vi "Game Controller.vi"(8 "error in (no error)":errorcluster, 9 "Direction":T1, 11 "Application in":refnum<class "Game.lvclass">) -> (0 "error out":errorcluster, 3 "Application out":refnum<class "Game.lvclass">)   [LabVIEW 2021, in "Game.lvclass"]
doc: "Handles the logic process to respawn, manage and control all elements that appear in the board game"
uses:
  Game.lvclass
  GameEl_class/private/Enum Direction.ctl
  Game.lvclass/Game.ctl
  Imposible_Snake_v2/LVApp/Modules/Sound Manager/Typedefs/Sound Effects.ctl
  Board Game_class/Board Game.lvclass
  Imposible_Snake_v2/LVApp/Modules/Sound Manager/Sound Manager.lvlib
  GameEl_class/GameEl.lvclass
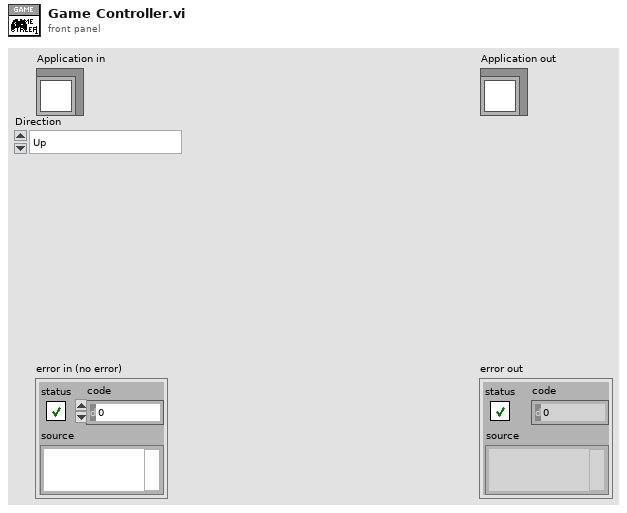
[diagram p1: front panel]
types:
  T1 = typedef "GameEl.lvclass/Enum Direction.ctl" = enum16{"Up", "Down", "Forward", "Backward"}
  T2 = typedef "Sound Manager.lvlib/Sound Effects.ctl" = enum16{"Bomb In", "Bomb Out", "Bomb Touched", "Game Over", "Victory", "Eat", "10 Fruits", "Eat2", "Eat3", "Eat4", "MaxShield", "Shield", "10p", "Grape In", "Grape Out", "20p", "30p", "40p", "50p", "60p", "70p", "80p", "90p", "100p", "All shields cracked", "Mouse In", "Mouse Out", "Mouse Eaten", "Grape Eaten", "States Recover", "Broken Shield", "Bonus", "Happy Time", "explode", "Game over musica", "Back Music", "Shield Catch", "Evil lough", "Cricket In", "Cricket eaten", "Lets Go", "Jump1", "Jump2", "Jump3", "Unstoppable", "Troll Music", "winner", "menu"}
  T3 = typedef "Game.lvclass/Packed Refs.ctl" = cluster{"graphics queue":refnum<queue>, "Stop Control Loop":refnum<user-event>, "Direction":refnum<notifier>, "Timer":refnum<data-value>}
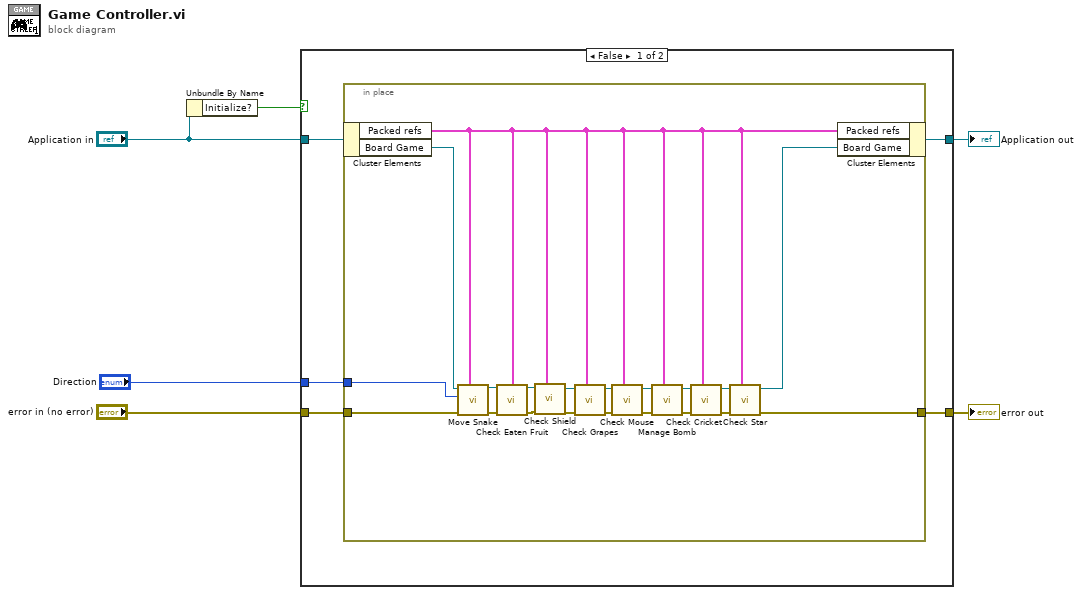
[diagram p0: block diagram]
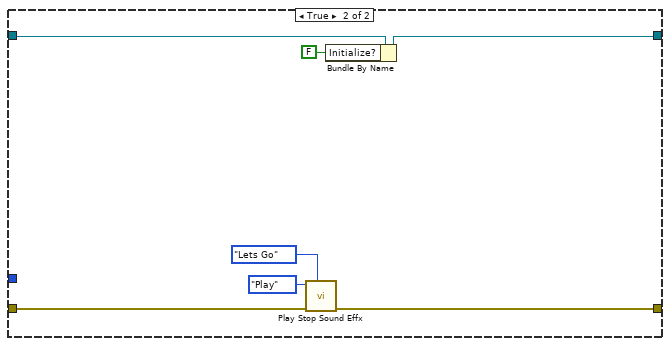
[diagram p2: hidden frame]
diagram:
  n1 = Unbundle By Name("Application in") -> ("Initialize?"=w1:bool)
  n2 = case shown="False" w1 {
    tunnel: "Application in" -> [w11 w38]
    tunnel: "error in (no error)" -> [w10 w32]
    tunnel: [w9 w33] -> w5
    tunnel: [w8 w37] -> w4
    tunnel: "Direction" -> [w7 _]
    frame False {
      n3 = in-place {
        in-place-border: w10 -> [w15]
        in-place-border: [w14] -> w9
        in-place-border: w7 -> [w12]
        n4 = in-place-cluster #1(w11) -> ("Packed refs"=w13:T3, "Board Game"=w17:refnum<class "Board Game.lvclass">)
        n5 = call "Move Snake.vi"("Packed refs"=w13, "error in (no error)"=w15, "Direction"=w12, "Board Game in"=w17) -> ("error out"=w20:errorcluster, "Board Game out"=w31:refnum<class "Board Game.lvclass">)  [unwired: 6 in]
        n6 = call "Check Eaten Fruit.vi"("Board Game in"=w31, "Packed refs"=w13, "error in (no error)"=w20) -> ("Board Game out"=w24:refnum<class "Board Game.lvclass">, "error out"=w22:errorcluster)  [unwired: 11 in]
        n7 = call "Check Shield.vi"("Packed refs"=w13, "error in (no error)"=w22, "Board Game in"=w24) -> ("error out"=w21:errorcluster, "Board Game out"=w23:refnum<class "Board Game.lvclass">)  [unwired: 7 in]
        n8 = call "Check Grapes.vi"("Packed refs"=w13, "error in (no error)"=w21, "Board Game in"=w23) -> ("error out"=w30:errorcluster, "Board Game out"=w29:refnum<class "Board Game.lvclass">)  [unwired: 7 in]
        n9 = call "Check Mouse.vi"("Packed refs"=w13, "error in (no error)"=w30, "Board Game in"=w29) -> ("error out"=w28:errorcluster, "Board Game out"=w27:refnum<class "Board Game.lvclass">)  [unwired: 7 in]
        n10 = call "Manage Bomb.vi"("Packed refs"=w13, "error in (no error)"=w28, "Board Game in"=w27) -> ("error out"=w25:errorcluster, "Board Game out"=w26:refnum<class "Board Game.lvclass">)  [unwired: 7 in]
        n11 = call "Check Cricket.vi"("Packed refs"=w13, "error in (no error)"=w25, "Board Game in"=w26) -> ("error out"=w19:errorcluster, "Board Game out"=w18:refnum<class "Board Game.lvclass">)  [unwired: 7 in]
        n12 = call "Check Star.vi"("Packed refs"=w13, "error in (no error)"=w19, "Board Game in"=w18) -> ("error out"=w14:errorcluster, "Board Game out"=w16:refnum<class "Board Game.lvclass">)  [unwired: 7 in]
        n13 = in-place-cluster #1("Packed refs"=w13, "Board Game"=w16) -> (w8:refnum<class "Game.lvclass">)
      }
    }
    frame True {
      n14 = call "Play Stop Sound Effx.vi"("Sound Effect"=Sound_Effects."Lets Go", "Error In"=w32, "Function"=enum16{"Play", "Stop"}."Play") -> ("error in (no error)"=w33:errorcluster)  [unwired: 8 in]
      n15 = Bundle By Name(cluster=w38, "Initialize?"=FALSE) -> (w37:refnum<class "Game.lvclass">)
    }
  }
  "error out" <- w5
  "Application out" <- w4
